vi "Write SCH Config Parameters to FPGA.vi"(8 "error in (no error)":errorcluster, 10 "FPGA Configuration Values":T1={"Ln2 Filter Size"=10, "VT Quench Tick Limit"=4000000, "VT Quench Volt Limit"=0.1000061035156, "Joint Tick Limit"=4000000, "Joint Volt Limit"=0.0002000033855438, "CoWound Volt Limit"=0.2000122070312, "CoWound Tick Limit"=4000000, "SC Bus Limit"=0.0004000067710876, "SC Bus Tick Limit"=4000000, "ResMag Tick Limit"=1000000, "DAQ Cycle Ticks"=4096, "Res Mag dI/dt Delay"=256, "dI/dT scaling"=38.14697265625, "Pressure Inlet Limit (BarA)"=6.0, "Bore Tube Volt Limit"=0.5999999940395, "Pressure Outlet Limit (BarA)"=5.0, "Activation Current (kA)"=0.5, "Dump Resistor Scale Factor"=204.7939999998, "Co-Wound Asymmetry Factor"=-0.0026654, "Co-Wound Scale Factor"=60.04379999638, "Layer Scale Factors"=[4.000479996204, 3.501155003905, 3.50127799809, 3.501155003905, 3.001561000943, 3.001561000943, 3.50005300343, 3.500664994121, 3.501155003905, 4.000159993768, 3.999679997563, 4.000159993768, 3.998879998922, 3.999520003796, 3.999679997563, 4.000320002437, 4.00096000731, 4.000640004873], "Fudge Factors"=[0.0486624, 0.0491151, -0.0418637, -0.0149169, 0.0726134, -0.0451977, -0.0032112, -0.0234927, -0.002501, 0.0285479, -0.0270486, 0.003522, 0.0059306, -0.0088003, -0.0297659, 0.0390219], "Joint Scale Factors"=[0.0002005249261856, 0.0002005249261856, 0.0002004057168961, 0.000200480222702, 0.0002004057168961, 0.0002007633447647, 0.0002006888389587, 0.0002006441354752], "SC Bus Scale"=[0.09999999403954, 0.09999999403954, 0.001000002026558, 0.001000002026558, 0.0002005249261856, 0.0002006441354752], "Pressure Scale Factor"=[1.723690003157, 1.723690003157, 1.723690003157, 1.723690003157], "# Consecutive Zeros Fault"=1000, "Digitize Convert Ticks"=200, "Digitize Reset Ticks"=400, "Convert Clock Ticks"=20, "Digitize Read Delay Ticks"=38, "Digitize # Bits"=16, "HTS Lead Tick Limit"=4000000, "Res Lead Tick Limit"=4000000, "HTS Lead Trip"=0.1500000059605, "Res Lead Limit"=0.001953125, "HTS Lead FRZ"=0.006999999284744, "HTS Lead Warn"=0.001000002026558, "Low Current (kA)"=0.04500000178814, "Low Current Ticks"=400000000, "Low Current Delay Factor"=100, "HTS Resistance (nOhm)"=[0.0, 0.0], "Ticks to Close Relief"=80000000, "All Breaker Tick Limit"=400000000, "HTS Offset (microV)"=[0.0, 0.0], "Delay Ticks Between Bkr Reset"=1200000000, "Breaker Reset Ticks"=400000000, "PS Enable Reset Ticks"=400000000, "Reset Digitizer Ticks"=400000000, "Pressure Inlet Cooldown Limit"=12.0, "Pressure Outlet Cooldown Limit"=10.0, "Notification Email"="sth@magnet.fsu.edu"} {"Pressure Outlet Cooldown Limit" format="%.5g"; "Pressure Inlet Cooldown Limit" format="%.5g"; "HTS Offset (microV)" format="%_6g"; "HTS Resistance (nOhm)" format="%_6g"; "HTS Lead Warn" format="%_6g"; "HTS Lead FRZ" format="%_6g"; "Res Lead Limit" format="%_6g"; "HTS Lead Trip" format="%_6g"; "Pressure Scale Factor" format="%_6g"; "Joint Scale Factors" format="%_6g"; "Fudge Factors" format="%.7g"; "Co-Wound Asymmetry Factor" format="%.8g"; "Activation Current (kA)" format="%_6g"; "Pressure Outlet Limit (BarA)" format="%.5g"; "Bore Tube Volt Limit" format="%_6g"; "Pressure Inlet Limit (BarA)" format="%.5g"; "dI/dT scaling" format="%.11g"; "SC Bus Limit" format="%_6g"; "Joint Volt Limit" format="%_6g"; "VT Quench Volt Limit" format="%.5g"}, 11 "Refnum in":T2) -> (0 "error out":errorcluster, 3 "Refnum out":T2)   [LabVIEW 2020]
doc: "Author: Scott Hannahs <sth@magnet.fsu.edu>\nCopyright 2018 Florida State University, All rights reserved."
uses:
  RT Controls/FPGA SCH Digitizer Ref.ctl
  SCH Data Controls/FPGA Configure Parameters.ctl
  RT Server Sub VIs/RT Host Globals.vi
  <vilib>/Utility/error.llb/Error Cluster From Error Code.vi
  <vilib>/rvi/errors/niLvFpgaAdjustHostInterfaceError.vi
  <vilib>/rvi/interface/nirviReadWriteControl/nirviReadWriteControl.xnode
  NiFpgaLv.dll
  <vilib>/rvi/interface/Simulation/niFpgaSimulationCallBeginRW.vi
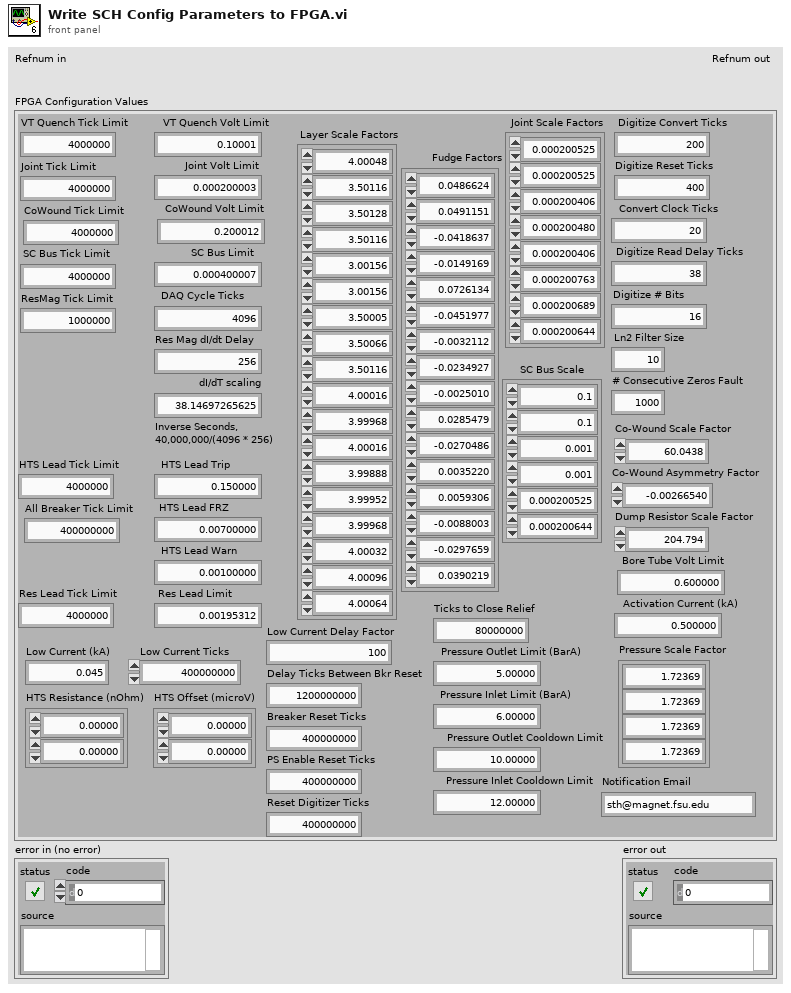
[diagram p1: front panel]
types:
  T1 = typedef "FPGA Configure Parameters.ctl" = cluster{"Ln2 Filter Size":i16, "VT Quench Tick Limit":u32, "VT Quench Volt Limit":dbl, "Joint Tick Limit":u32, "Joint Volt Limit":dbl, "CoWound Volt Limit":dbl, "CoWound Tick Limit":u32, "SC Bus Limit":dbl, "SC Bus Tick Limit":u32, "ResMag Tick Limit":u32, "DAQ Cycle Ticks":u32, "Res Mag dI/dt Delay":u32, "dI/dT scaling":dbl, "Pressure Inlet Limit (BarA)":dbl, "Bore Tube Volt Limit":dbl, "Pressure Outlet Limit (BarA)":dbl, "Activation Current (kA)":dbl, "Dump Resistor Scale Factor":dbl, "Co-Wound Asymmetry Factor":dbl, "Co-Wound Scale Factor":dbl, "Layer Scale Factors":dbl[], "Fudge Factors":dbl[], "Joint Scale Factors":dbl[], "SC Bus Scale":dbl[], "Pressure Scale Factor":dbl[], "# Consecutive Zeros Fault":i16, "Digitize Convert Ticks":u32, "Digitize Reset Ticks":u32, "Convert Clock Ticks":u32, "Digitize Read Delay Ticks":u32, "Digitize # Bits":u32, "HTS Lead Tick Limit":u32, "Res Lead Tick Limit":u32, "HTS Lead Trip":dbl, "Res Lead Limit":dbl, "HTS Lead FRZ":dbl, "HTS Lead Warn":dbl, "Low Current (kA)":dbl, "Low Current Ticks":u32, "Low Current Delay Factor":u16, "HTS Resistance (nOhm)":dbl[], "Ticks to Close Relief":u32, "All Breaker Tick Limit":u32, "HTS Offset (microV)":dbl[], "Delay Ticks Between Bkr Reset":u32, "Breaker Reset Ticks":u32, "PS Enable Reset Ticks":u32, "Reset Digitizer Ticks":u32, "Pressure Inlet Cooldown Limit":dbl, "Pressure Outlet Cooldown Limit":dbl, "Notification Email":string}
  T2 = typedef "FPGA SCH Digitizer Ref.ctl" = refnum<k20>
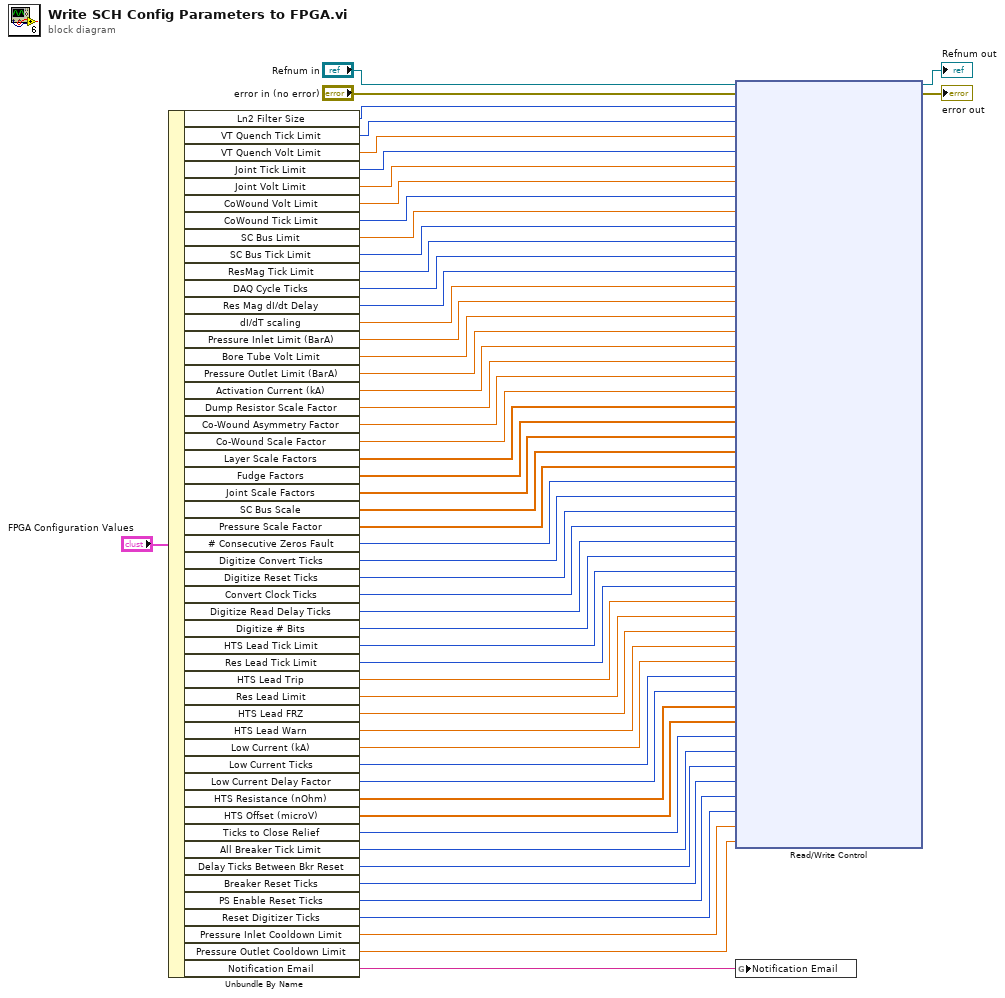
[diagram p0: block diagram]
diagram:
  n1 = Unbundle By Name("FPGA Configuration Values") -> ("Ln2 Filter Size"=w51:i16, "VT Quench Tick Limit"=w50:u32, "VT Quench Volt Limit"=w49:dbl, "Joint Tick Limit"=w48:u32, "Joint Volt Limit"=w47:dbl, "CoWound Volt Limit"=w46:dbl, "CoWound Tick Limit"=w45:u32, "SC Bus Limit"=w44:dbl, "SC Bus Tick Limit"=w43:u32, "ResMag Tick Limit"=w42:u32, "DAQ Cycle Ticks"=w41:u32, "Res Mag dI/dt Delay"=w40:u32, "dI/dT scaling"=w39:dbl, "Pressure Inlet Limit (BarA)"=w38:dbl, "Bore Tube Volt Limit"=w37:dbl, "Pressure Outlet Limit (BarA)"=w36:dbl, "Activation Current (kA)"=w35:dbl, "Dump Resistor Scale Factor"=w34:dbl, "Co-Wound Asymmetry Factor"=w33:dbl, "Co-Wound Scale Factor"=w32:dbl, "Layer Scale Factors"=w31:dbl[], "Fudge Factors"=w30:dbl[], "Joint Scale Factors"=w29:dbl[], "SC Bus Scale"=w28:dbl[], "Pressure Scale Factor"=w27:dbl[], "# Consecutive Zeros Fault"=w26:i16, "Digitize Convert Ticks"=w25:u32, "Digitize Reset Ticks"=w24:u32, "Convert Clock Ticks"=w23:u32, "Digitize Read Delay Ticks"=w22:u32, "Digitize # Bits"=w21:u32, "HTS Lead Tick Limit"=w20:u32, "Res Lead Tick Limit"=w19:u32, "HTS Lead Trip"=w18:dbl, "Res Lead Limit"=w17:dbl, "HTS Lead FRZ"=w16:dbl, "HTS Lead Warn"=w15:dbl, "Low Current (kA)"=w14:dbl, "Low Current Ticks"=w13:u32, "Low Current Delay Factor"=w12:u16, "HTS Resistance (nOhm)"=w11:dbl[], "HTS Offset (microV)"=w9:dbl[], "Ticks to Close Relief"=w10:u32, "All Breaker Tick Limit"=w8:u32, "Delay Ticks Between Bkr Reset"=w7:u32, "Breaker Reset Ticks"=w6:u32, "PS Enable Reset Ticks"=w5:u32, "Reset Digitizer Ticks"=w4:u32, "Pressure Inlet Cooldown Limit"=w3:dbl, "Pressure Outlet Cooldown Limit"=w2:dbl, "Notification Email"=w1:string)
  n2 = xnode "Read/Write Control"("FPGA VI Reference In"="Refnum in", "error in"="error in (no error)", "Ln2 Filter Size"=w51, "VT Quench Tick Limit"=w50, "VT Quench Volt Limit"=w49, "Joint Tick Limit"=w48, "Joint Volt Limit"=w47, "CoWound Volt Limit"=w46, "CoWound Tick Limit"=w45, "SC Bus Limit"=w44, "SC Bus Tick Limit"=w43, "ResMag Tick Limit"=w42, "DAQ Cycle Ticks"=w41, "Res Mag dI/dt Delay"=w40, "dI/dT scaling"=w39, "Pressure Inlet Limit (BarA)"=w38, "Bore Tube Volt Limit"=w37, "Pressure Outlet Limit (BarA)"=w36, "Activation Current (kA)"=w35, "Dump Resistor Scale Factor"=w34, "Co-Wound Asymmetry Factor"=w33, "Co-Wound Scale Factor"=w32, "Layer Scale Factors"=w31, "Fudge Factors"=w30, "Joint Scale Factors"=w29, "SC Bus Scale"=w28, "Pressure Scale Factor"=w27, "# Consecutive Zeros Fault"=w26, "Digitize Convert Ticks"=w25, "Digitize Reset Ticks"=w24, "Convert Clock Ticks"=w23, "Digitize Read Delay Ticks"=w22, "Digitize # Bits"=w21, "HTS Lead Tick Limit"=w20, "Res Lead Tick Limit"=w19, "HTS Lead Trip"=w18, "Res Lead Limit"=w17, "HTS Lead FRZ"=w16, "HTS Lead Warn"=w15, "Low Current (kA)"=w14, "Low Current Ticks"=w13, "Low Current Delay Factor"=w12, "HTS Resistance (nOhm)"=w11, "HTS Offset (microV)"=w9, "Ticks to Close Relief"=w10, "All Breaker Tick Limit"=w8, "Delay Ticks Between Bkr Reset"=w7, "Breaker Reset Ticks"=w6, "PS Enable Reset Ticks"=w5, "Reset Digitizer Ticks"=w4, "Pressure Inlet Cooldown Limit"=w3, "Pressure Outlet Cooldown Limit"=w2) -> ("FPGA VI Reference Out"=→"Refnum out":T2, "error out"=→"error out":errorcluster)
  n3 = global write "RT Host Globals.vi" "Notification Email"(w1) -> ()
